vi "recursive2.vi"() -> ()   [LabVIEW 2014]
uses:
  <vilib>/LabVIEW Targets/FPGA/cRIO/shared/nicrio_ModuleControls/nicrio_cRIO-9467_Altitude.ctl
  <vilib>/LabVIEW Targets/FPGA/cRIO/shared/nicrio_ModuleControls/nicrio_cRIO-9467_Longitude.ctl
  <vilib>/LabVIEW Targets/FPGA/cRIO/shared/nicrio_ModuleControls/nicrio_cRIO-9467_Latitude.ctl
  <vilib>/LabVIEW Targets/FPGA/cRIO/shared/nicrio_ModuleControls/nicrio_cRIO-9225_DataRatesRing.ctl
  <vilib>/LabVIEW Targets/FPGA/cRIO/shared/nicrio_ModuleControls/nicrio_cRIO-9227_DataRatesRing.ctl
  <vilib>/rvi/FXPMathLib/FxpSinAndCos/subVIs/nifxpmath_SinAndCos_SimConfig.ctl
  <vilib>/rvi/FXPMathLib/FxpRectToPolar/subVIs/nifxpmath_RectToPolar_SimConfig.ctl
  <vilib>/rvi/Emulation/niFpgaGetClockAttributes.vi
  <vilib>/rvi/Emulation/niFpgaSctlEmulationGetInTimedLoop.vi
  <vilib>/rvi/Emulation/niFpgaEmulationReportErrorSimple.vi
  <vilib>/rvi/eio/common/nirviEmuTemplateMethod_errors.vi
  <vilib>/rvi/eio/common/nirviEmuTemplatePropertyGet_noerrors.vi
  <vilib>/rvi/Emulation/niFpgaCriticalErrorInLSC.vi
  <vilib>/rvi/Memory/Memory_Emulation/nirvimemoryFastEmulation.vi
  <vilib>/rvi/Memory/Memory_Emulation/nirvimemoryEmulation.vi
  <vilib>/rvi/Emulation/niFpgaEmulationIsFPGAContextNoSignature.vi
  <vilib>/rvi/DataTransferAndStorage/Container/Common/niFpgaContainerGetUniqueNameForEmu.vi
  <vilib>/rvi/Emulation/niFpgaProcessEmulError.vi
  <vilib>/rvi/errors/nirviReportUnexpectedCaseInternalError (U32).vi
  <vilib>/rvi/FXPMathLib/FxpSinAndCos/simVIs/DllFxpSinAndCosTemp_sub.vi
  <vilib>/rvi/FXPMathLib/FxpRectToPolar/simVIs/DllFxpRectToPolarTemp_sub.vi
  <vilib>/rvi/eio/common/nirviEmuTemplatePropertySet_noerrors.vi
  <vilib>/rvi/DataTransferAndStorage/Container/Common/niFpgaContainerSetEmuInfo.vi
  <vilib>/rvi/eio/common/nirviEmuReportErrorAndStop.vi
  <vilib>/rvi/eio/common/nirviEmuTemplatePropertyGet_errors.vi
  <vilib>/eio/EIOMethodNode/EIOMethodNode.xnode
  <vilib>/eio/EIOPropertyNode/EIOPropertyNode.xnode
  <vilib>/eio/EIONode/EIONode.xnode
  <vilib>/rvi/DataTransferAndStorage/Container/XNode/niFpgaContainer.xnode
  <vilib>/rvi/FXPMathLib/FxpMul/XNode/nifxpmath_Multiplier.xnode
  <vilib>/rvi/FXPMathLib/FxpSinAndCos/XNode/nifxpmath_SinAndCos.xnode
  <vilib>/rvi/FXPMathLib/FxpAdd/XNode/nifxpmath_Add.xnode
  <vilib>/rvi/FXPMathLib/FxpRectToPolar/XNode/nifxpmath_RectToPolar.xnode
  <vilib>/rvi/FXPMathLib/FxpSub/XNode/nifxpmath_Sub.xnode
  <vilib>/rvi/LocalResourceManager/LocalResourceManager.xnode
  <vilib>/rvi/FXPMathLib/sim/FxpSim.dll
  <vilib>/rvi/eio/common/nirviEmuTemplatePropertySet_errors.vi
  fpga timekeeper/FPGA Timekeeper.lvlib
panel:
  out "FPGA Timekeeper time (ns) 2":u64
  out "GPS status":T1(ring)
  out "FPGA Timekeeper locked":bool
  out "offset from time reference":i32
  out "antenna status":T2(ring)
  out "satellites available":u8
  out "UTC offset":i8
  out "UTC offset valid":bool
  out "Firmware Version":u32 format="%.0x"
  out "Vendor ID":u16 format="%.0x"
  out "Module ID":u16 format="%.0x"
  out "Serial Number":u32 format="%.0x"
  out "FPGA Error Out":errorcluster
  in  "stop 2":bool
  out "PPS Timestamp (TAI)":u64
  out "UTC Offset":i8
  out "UTC Offset Valid":bool
  out "GPS Status":T1(ring)
  out "Antenna Status":T2(ring)
  out "Leap Second Direction":enum8{"Add", "Delete"}(ring)
  out "Leap Second Pending":bool
  out "Leap Second Occurred":bool
  out "Satellites Available":u8
  out "Self-Survey Complete":bool
  out "Latitude (°)":T3 format="%.6f"
  out "Longitude (°)":T4 format="%.6g"
  out "Altitude (m)":T5 format="%.2f"
  out "Timed Out":bool
  out "Iterations":i32
  out "ROCOF":fxp<+/-,17,17>
  out "current frequency":fxp<+/-,35,18>
  out "Voltage Frequency":fxp<+/-,35,18>
  out "magnitude":fxp<+,62,19>[](array[numeric])
  out "phase angle":fxp<+/-,22,10>[](array[numeric])
  out "Array":T6(array[cluster])
  out "r":fxp<+,60,17>[](array[numeric])
  out "theta":fxp<+/-,22,10>[](array[numeric])
  in  "stop":bool
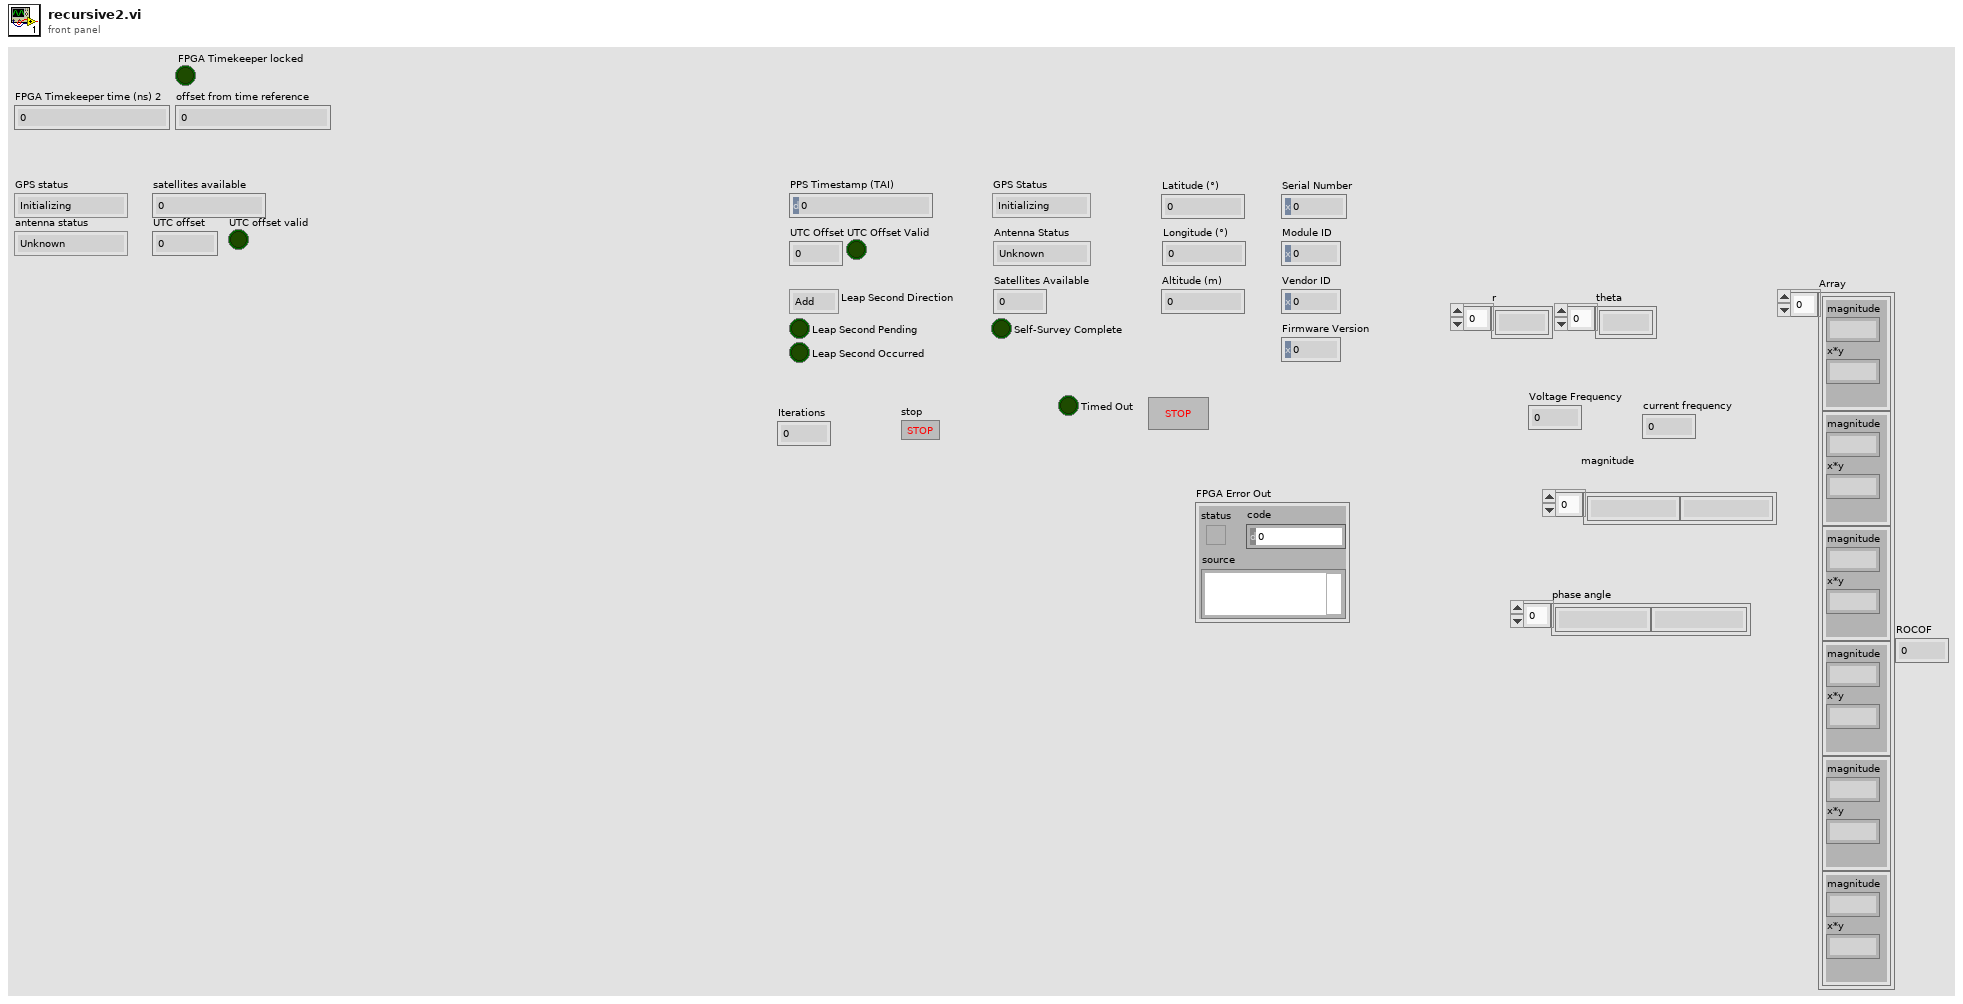
[diagram p1: front panel]
types:
  T1 = enum8{"Initializing", "Normal", "Unable to get fix"}
  T2 = enum8{"Unknown", "Normal", "Absent", "Overcurrent"}
  T3 = typedef "nicrio_cRIO-9467_Latitude.ctl" = fxp<+/-,28,8>
  T4 = typedef "nicrio_cRIO-9467_Longitude.ctl" = fxp<+/-,29,9>
  T5 = typedef "nicrio_cRIO-9467_Altitude.ctl" = fxp<+/-,24,17>
  T6 = cluster{"magnitude":fxp<+,62,19>, "x*y":fxp<+/-,22,10>}[]
  T7 = typedef "nicrio_cRIO-9227_DataRatesRing.ctl" = u8
  T8 = typedef "nicrio_cRIO-9225_DataRatesRing.ctl" = u8
  T9 = cluster{"magnitude":fxp<+,62,19>, "x*y":fxp<+/-,22,10>}
  T10 = cluster{"magnitude":fxp<+,60,17>, "x*y":fxp<+/-,22,10>}
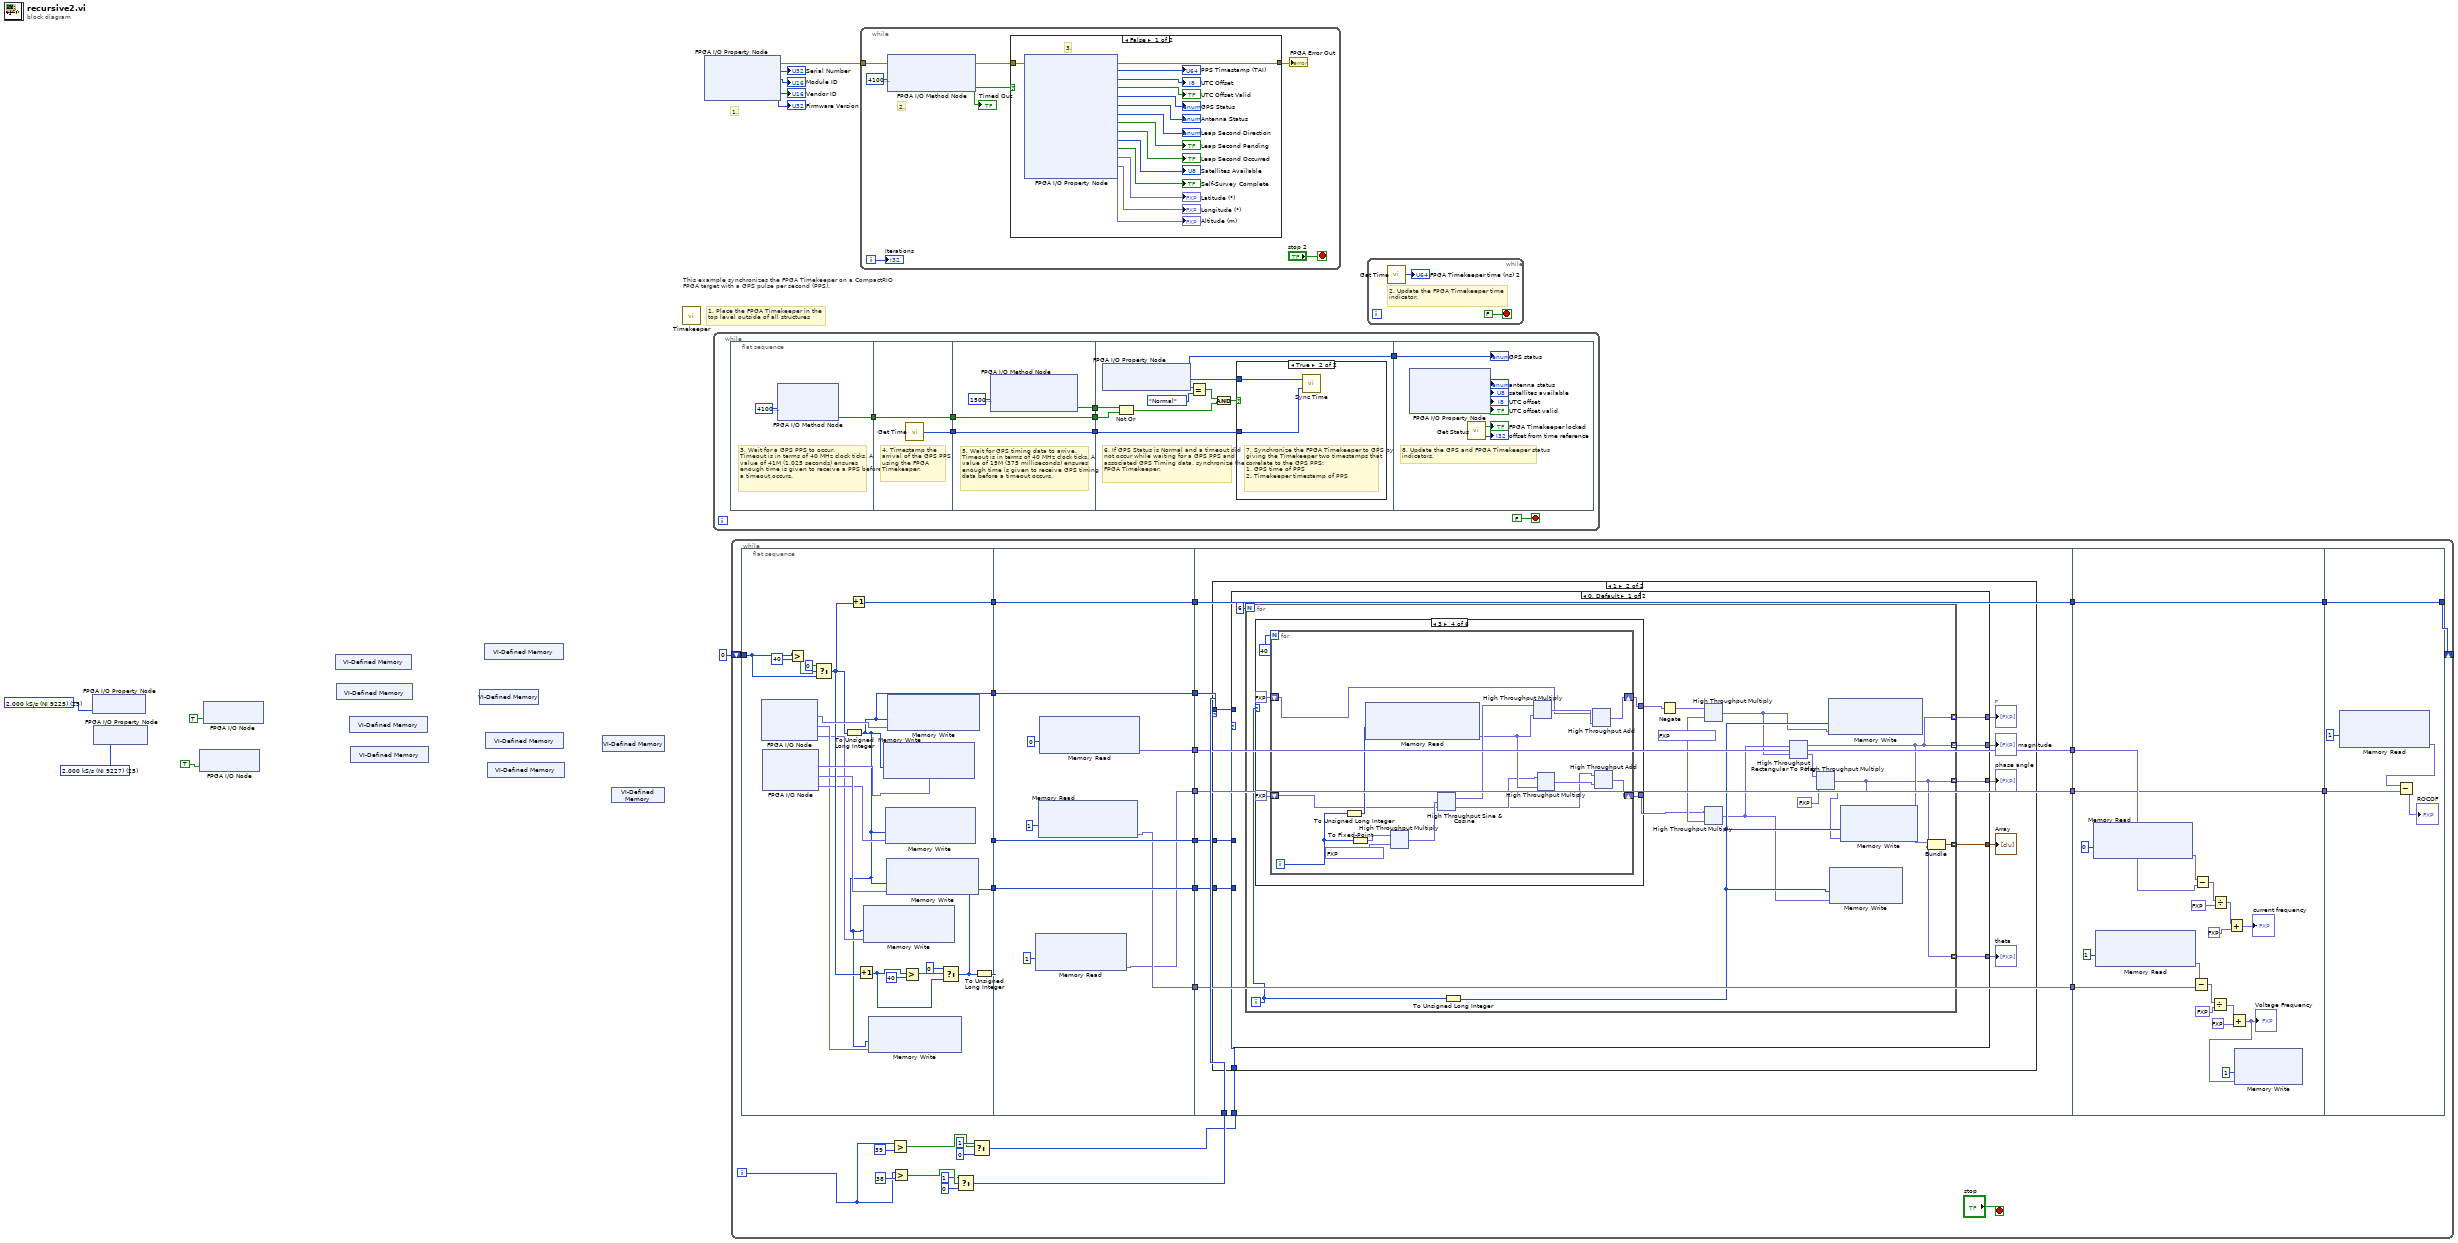
[diagram p0: block diagram]
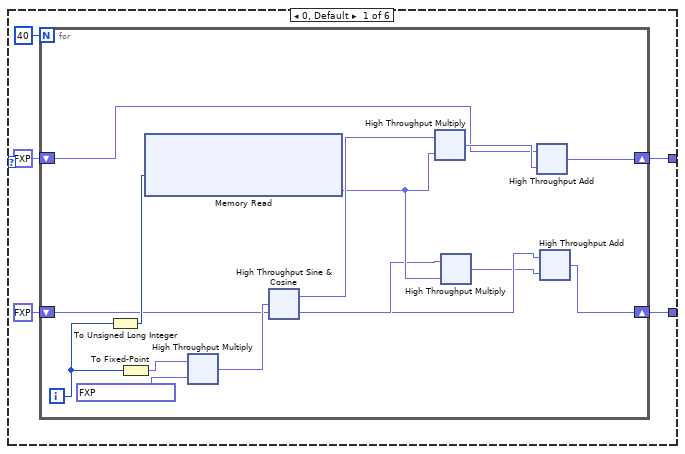
[diagram p5: hidden frame]
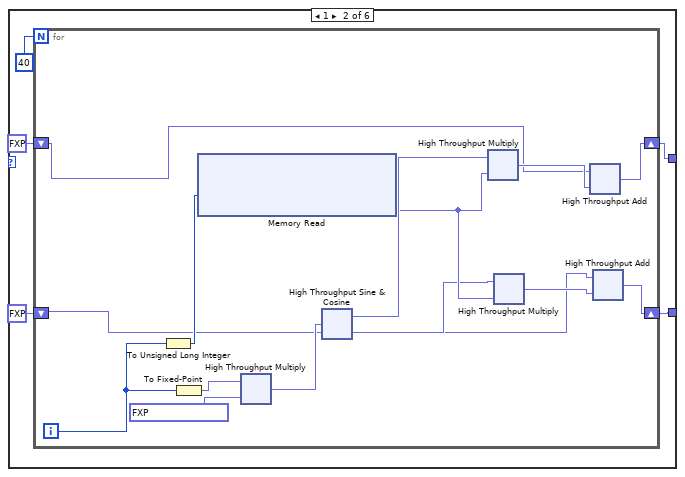
[diagram p6: hidden frame]
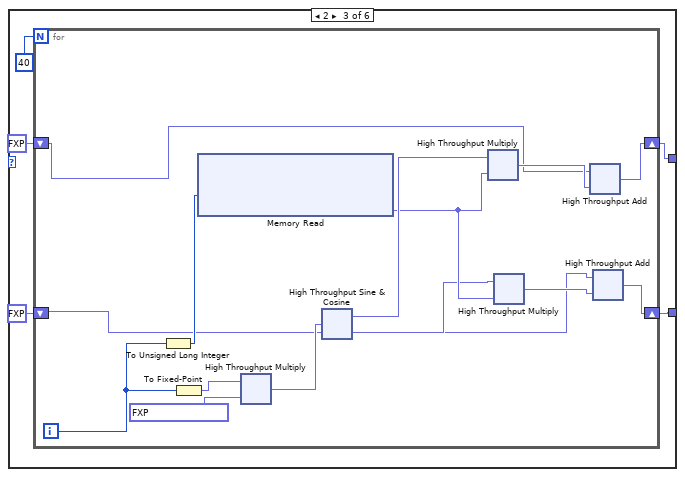
[diagram p7: hidden frame]
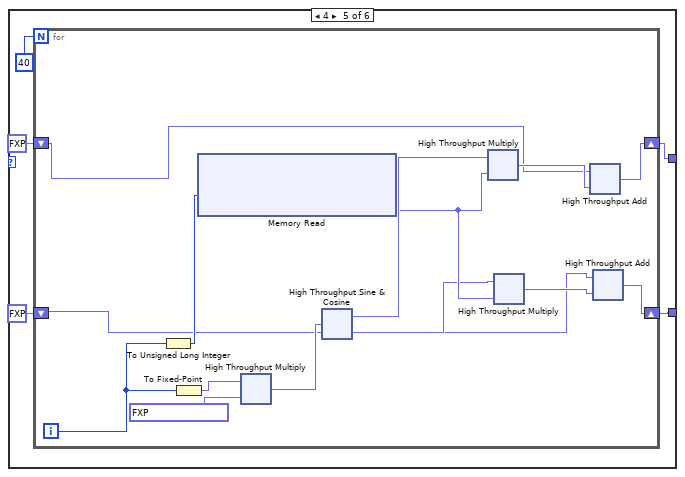
[diagram p8: hidden frame]
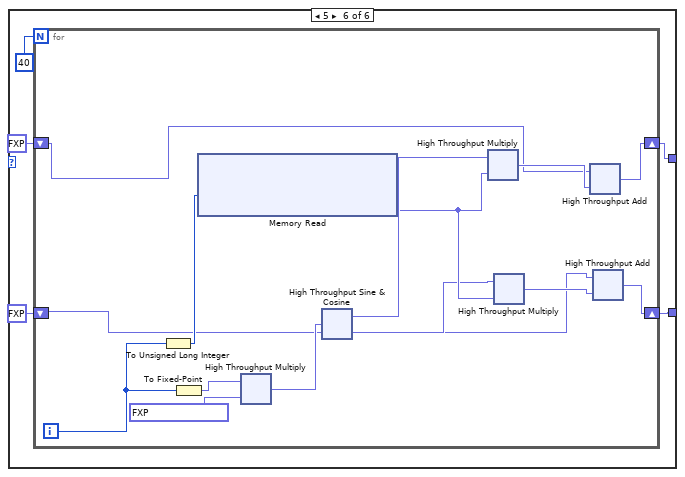
[diagram p9: hidden frame]
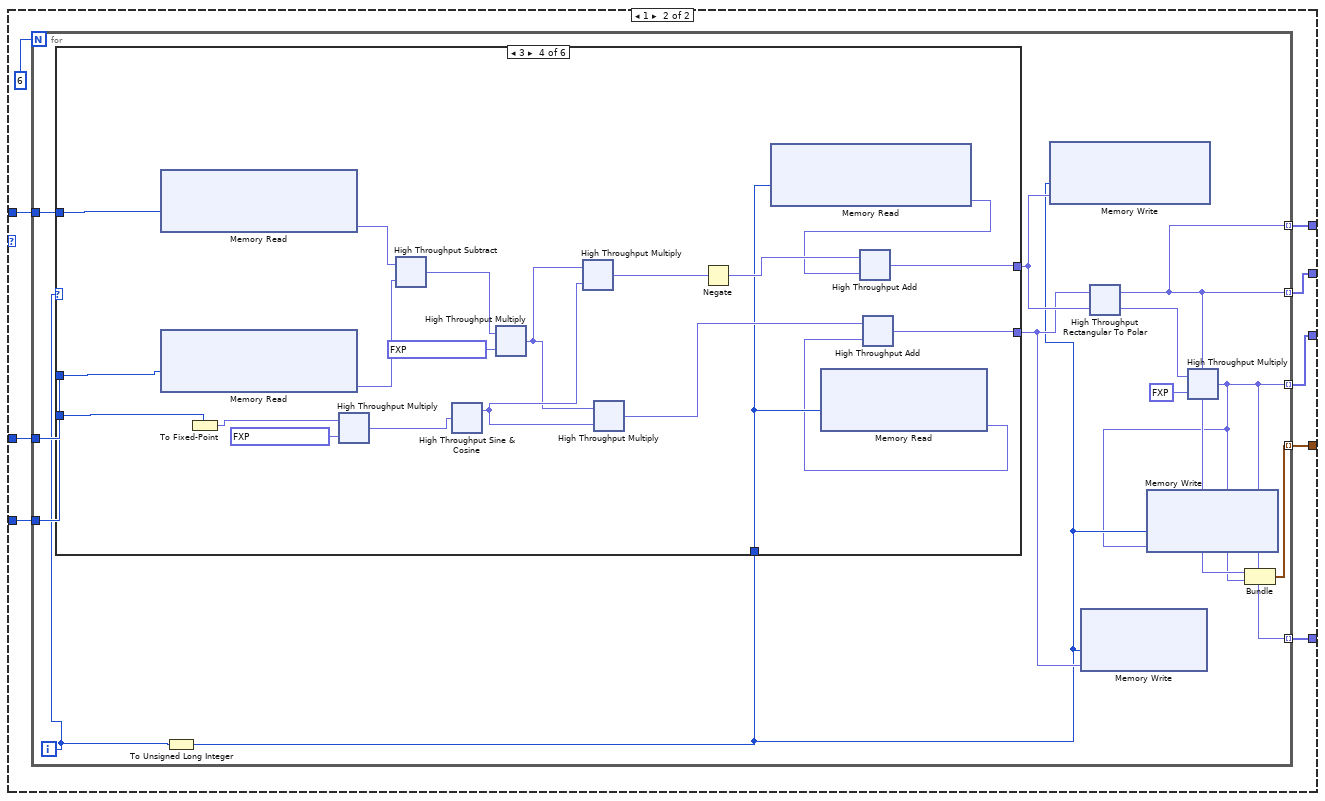
[diagram p10: hidden frame]
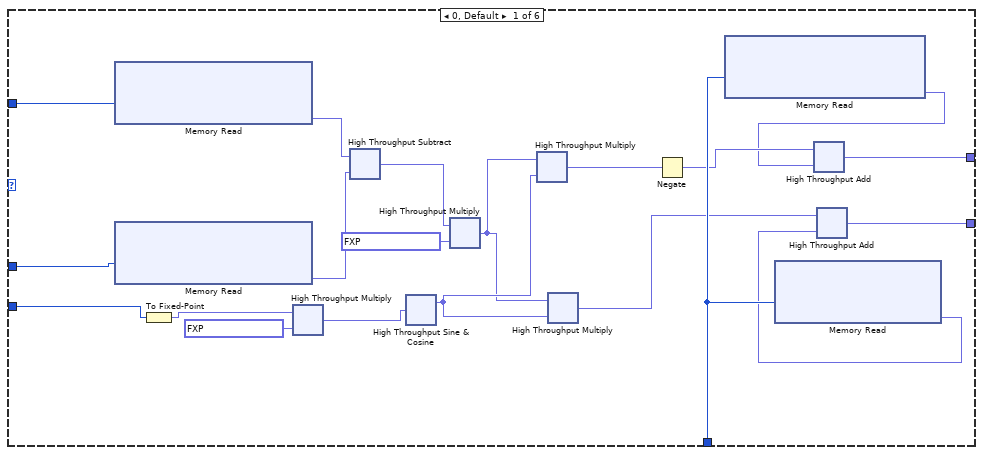
[diagram p11: hidden frame]
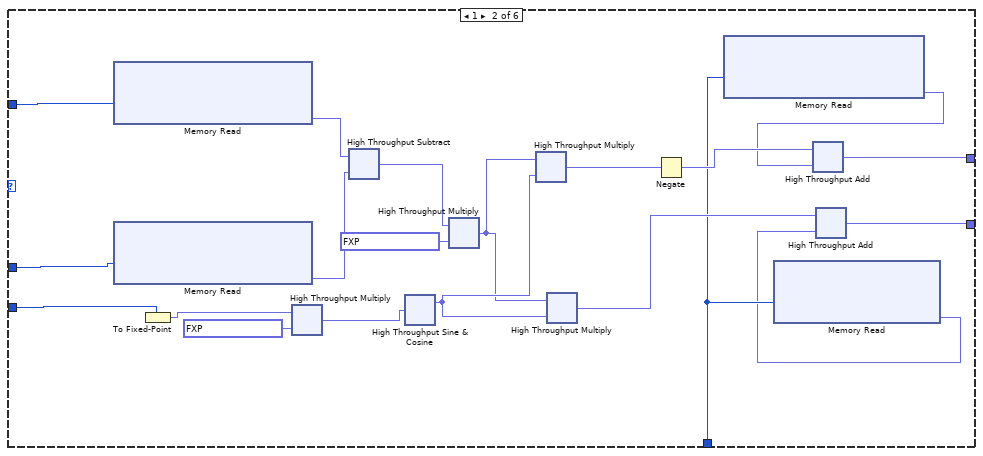
[diagram p12: hidden frame]
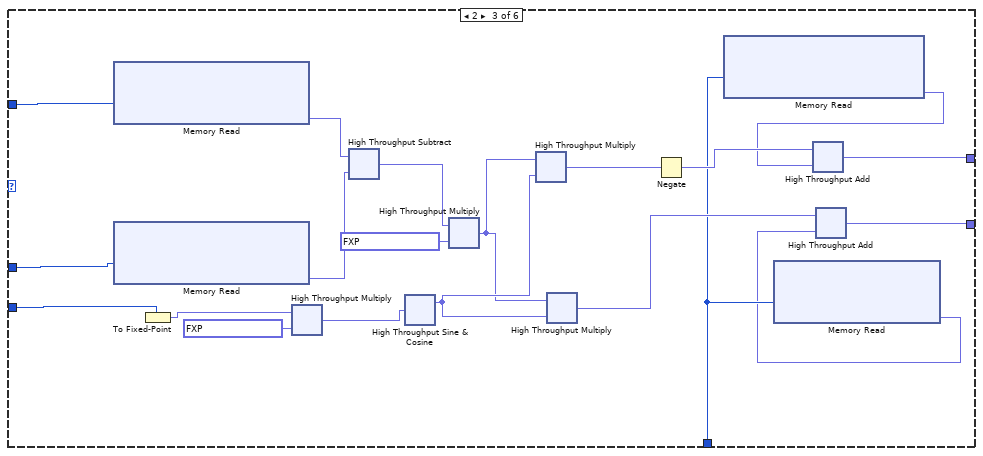
[diagram p13: hidden frame]
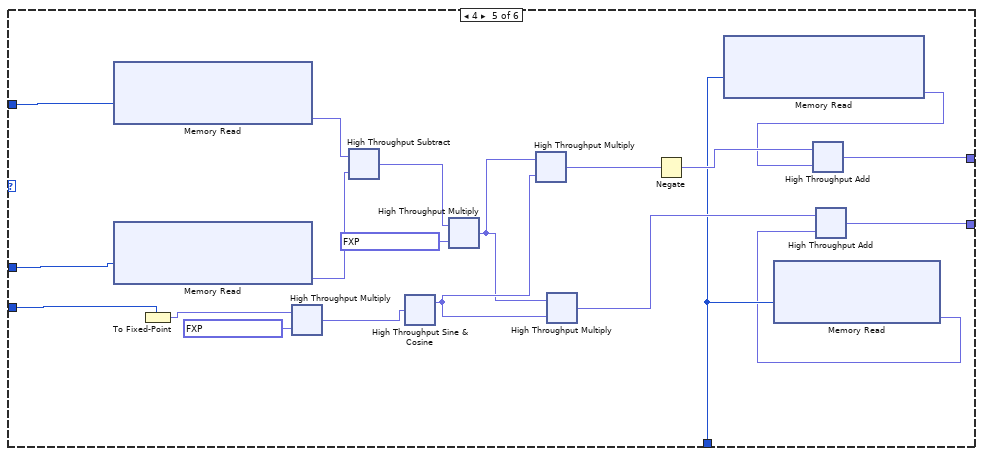
[diagram p14: hidden frame]
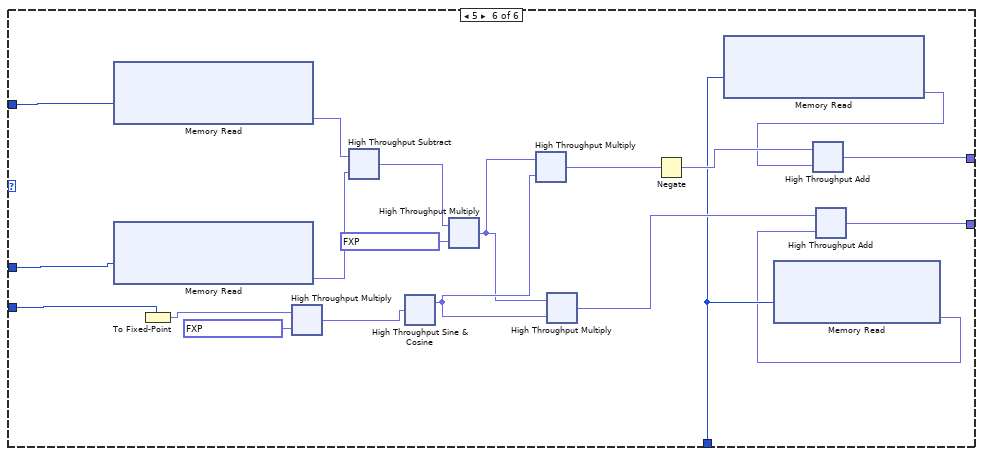
[diagram p15: hidden frame]
diagram:
  w10 = T7 25 items=["50.000 kS/s (NI 9227)"=1, "25.000 kS/s (NI 9227)"=2, "16.667 kS/s (NI 9227)"=3, "12.500 kS/s (NI 9227)"=4, "10.000 kS/s (NI 9227)"=5, "8.333 kS/s (NI 9227)"=6, "7.143 kS/s (NI 9227)"=7, "6.250 kS/s (NI 9227)"=8, "5.556 kS/s (NI 9227)"=9, "5.000 kS/s (NI 9227)"=10, "4.545 kS/s (NI 9227)"=11, "4.167 kS/s (NI 9227)"=12, "3.846 kS/s (NI 9227)"=13, "3.571 kS/s (NI 9227)"=14, "3.333 kS/s (NI 9227)"=15, "3.125 kS/s (NI 9227)"=16, "2.941 kS/s (NI 9227)"=17, "2.778 kS/s (NI 9227)"=18, "2.632 kS/s (NI 9227)"=19, "2.500 kS/s (NI 9227)"=20, "2.381 kS/s (NI 9227)"=21, "2.273 kS/s (NI 9227)"=22, "2.174 kS/s (NI 9227)"=23, "2.083 kS/s (NI 9227)"=24, "2.000 kS/s (NI 9227)"=25, "1.923 kS/s (NI 9227)"=26, "1.852 kS/s (NI 9227)"=27, "1.786 kS/s (NI 9227)"=28, "1.724 kS/s (NI 9227)"=29, "1.667 kS/s (NI 9227)"=30, "1.613 kS/s (NI 9227)"=31] ("Data Rate")
  w7 = T8 25 items=["50.000 kS/s (NI 9225)"=1, "25.000 kS/s (NI 9225)"=2, "16.667 kS/s (NI 9225)"=3, "12.500 kS/s (NI 9225)"=4, "10.000 kS/s (NI 9225)"=5, "8.333 kS/s (NI 9225)"=6, "7.143 kS/s (NI 9225)"=7, "6.250 kS/s (NI 9225)"=8, "5.556 kS/s (NI 9225)"=9, "5.000 kS/s (NI 9225)"=10, "4.545 kS/s (NI 9225)"=11, "4.167 kS/s (NI 9225)"=12, "3.846 kS/s (NI 9225)"=13, "3.571 kS/s (NI 9225)"=14, "3.333 kS/s (NI 9225)"=15, "3.125 kS/s (NI 9225)"=16, "2.941 kS/s (NI 9225)"=17, "2.778 kS/s (NI 9225)"=18, "2.632 kS/s (NI 9225)"=19, "2.500 kS/s (NI 9225)"=20, "2.381 kS/s (NI 9225)"=21, "2.273 kS/s (NI 9225)"=22, "2.174 kS/s (NI 9225)"=23, "2.083 kS/s (NI 9225)"=24, "2.000 kS/s (NI 9225)"=25, "1.923 kS/s (NI 9225)"=26, "1.852 kS/s (NI 9225)"=27, "1.786 kS/s (NI 9225)"=28, "1.724 kS/s (NI 9225)"=29, "1.667 kS/s (NI 9225)"=30, "1.613 kS/s (NI 9225)"=31] ("Data Rate")
  # "This example synchronizes the FPGA Timekeeper on a CompactRIO FPGA target with a GPS pulse per second (PPS)."
  # "1. Place the FPGA Timekeeper in the\ntop level outside of all structures"
  # "1."
  n1 = xnode "FPGA I/O Property Node"("Data Rate"=w7) -> ()  [unwired: 1 in, 1 out]
  n2 = xnode "FPGA I/O Property Node"("Data Rate"=w10) -> ()  [unwired: 1 in, 1 out]
  n3 = xnode "FPGA I/O Node"("Mod2/Start"=TRUE) -> ()  [unwired: 1 in, 1 out]
  n4 = xnode "FPGA I/O Node"("Mod1/Start"=TRUE) -> ()  [unwired: 1 in, 1 out]
  n5 = xnode "VI-Defined Memory"() -> ()  [unwired: 1 out]
  n6 = xnode "VI-Defined Memory"() -> ()  [unwired: 1 out]
  n7 = xnode "VI-Defined Memory"() -> ()  [unwired: 1 out]
  n8 = xnode "VI-Defined Memory"() -> ()  [unwired: 1 out]
  n9 = xnode "VI-Defined Memory"() -> ()  [unwired: 1 out]
  n10 = xnode "VI-Defined Memory"() -> ()  [unwired: 1 out]
  n11 = xnode "VI-Defined Memory"() -> ()  [unwired: 1 out]
  n12 = xnode "VI-Defined Memory"() -> ()  [unwired: 1 out]
  n13 = xnode "VI-Defined Memory"() -> ()  [unwired: 1 out]
  n14 = xnode "VI-Defined Memory"() -> ()  [unwired: 1 out]
  n15 = call "Timekeeper.vi"() -> ()  [unwired: 12 in]
  n16 = xnode "FPGA I/O Property Node"() -> ("error out"=w1:errorcluster, "Serial Number"=→"Serial Number":u32, "Module ID"=→"Module ID":u16, "Vendor ID"=→"Vendor ID":u16, "Firmware Version"=→"Firmware Version":u32)  [unwired: 2 in, 1 out]
  n17 = while {
    stop <- FALSE stop-if-true
    n18 = flat-sequence {
      tunnel: [w19] -> w17
      tunnel: w17 -> [w22]
      tunnel: [w22] -> w16
      tunnel: [w21] -> w14
      tunnel: [w25] -> w18
      tunnel: w16 -> [w24]
      tunnel: [w24] -> w15
      tunnel: w14 -> [w23]
      tunnel: [w23] -> w13
      tunnel: w18 -> [w34]
      tunnel: w15 -> [w33]
      tunnel: w13 -> [w28]
      tunnel: [w27] -> w12
      tunnel: w12 -> [w44]
      frame #0 {
        # "3. Wait for a GPS PPS to occur.\nTimeout is in terms of 40 MHz clock ticks. A value of 41M (1.025 seconds) ensures enough time is given to receive a PPS before a timeout occurs."
        n19 = xnode "FPGA I/O Method Node"("Timeout"=41000000) -> ("Timed Out"=w19:bool)  [unwired: 1 in, 1 out]
      }
      frame #1 {
        # "4. Timestamp the arrival of the GPS PPS using the FPGA Timekeeper."
        n20 = call "Get Time.vi"() -> ("time (ns)"=w21:u64)
      }
      frame #2 {
        # "5. Wait for GPS timing data to arrive.\nTimeout is in terms of 40 MHz clock ticks. A value of 15M (375 milliseconds) ensures enough time is given to receive GPS timing data before a timeout occurs."
        n21 = xnode "FPGA I/O Method Node"("Timeout"=15000000) -> ("Timed Out"=w25:bool)  [unwired: 1 in, 1 out]
      }
      frame #3 {
        # "6. If GPS Status is Normal and a timeout did not occur while waiting for a GPS PPS and associated GPS Timing data, synchronize the FPGA Timekeeper."
        n22 = xnode "FPGA I/O Property Node"() -> ("PPS Timestamp (TAI)"=w29:u64, "GPS Status"=w27:T1)  [unwired: 1 in, 1 out]
        n23 = Not Or(1:w33, 2:w34) -> (0:w31:bool)
        n24 = Equal?(x=w27, y=T1."Normal") -> (x = y?=w32:bool)
        n25 = And(x=w32, y=w31) -> (x .and. y?=w30:bool)
        n26 = case shown="True" w30 {
          tunnel: w29 -> [_ w37]
          tunnel: w28 -> [_ w36]
          frame False {
          }
          frame True {
            # "7. Synchronize the FPGA Timekeeper to GPS by giving the Timekeeper two timestamps that correlate to the GPS PPS:\n1. GPS time of PPS\n2. Timekeeper timestamp of PPS"
            n27 = call "Sync Time.vi"("FPGA Timekeeper time (ns)"=w36, "time reference time (ns)"=w37) -> ()
          }
        }
      }
      frame #4 {
        # "8. Update the GPS and FPGA Timekeeper status indicators."
        n28 = xnode "FPGA I/O Property Node"() -> ("Antenna Status"=→"antenna status":T2, "Satellites Available"=→"satellites available":u8, "UTC Offset"=→"UTC offset":i8, "UTC Offset Valid"=→"UTC offset valid":bool)  [unwired: 1 in, 1 out]
        n29 = call "Get Status.vi"() -> ("FPGA Timekeeper locked"=→"FPGA Timekeeper locked":bool, "offset from time reference"=→"offset from time reference":i32)
        "GPS status" <- w44
      }
    }
  }
  n30 = while {
    shift-right: [w74] -> _
    shift-left: i16 0 -> [w75]
    i -> [w64]
    stop <- "stop" stop-if-true
    n31 = flat-sequence {
      tunnel: w75 -> [w90]
      tunnel: [w89] -> w60
      tunnel: [w76] -> w58
      tunnel: [w82] -> w56
      tunnel: [w81] -> w54
      tunnel: w60 -> [w104]
      tunnel: [w104] -> w59
      tunnel: w58 -> [w103]
      tunnel: [w103] -> w57
      tunnel: w56 -> [w102]
      tunnel: [w102] -> w55
      tunnel: w54 -> [w101]
      tunnel: [w101] -> w53
      tunnel: [w98] -> w51
      tunnel: [w97] -> w50
      tunnel: [w95] -> w47
      tunnel: w59 -> [w113]
      tunnel: w70 -> [w112]
      tunnel: w67 -> [w111]
      tunnel: w57 -> [w110]
      tunnel: w55 -> [w109]
      tunnel: w53 -> [w108]
      tunnel: [w113] -> w61
      tunnel: [w107] -> w52
      tunnel: w51 -> [w107]
      tunnel: w50 -> [w106]
      tunnel: [w106] -> w49
      tunnel: w47 -> [w105]
      tunnel: [w105] -> w46
      tunnel: w61 -> [w849]
      tunnel: w52 -> [w844]
      tunnel: w49 -> [w843]
      tunnel: [w849] -> w48
      tunnel: w46 -> [w831]
      tunnel: [w831] -> w45
      tunnel: [w854] -> w74
      tunnel: w48 -> [w854]
      tunnel: w45 -> [w851]
      frame #0 {
        n32 = xnode "FPGA I/O Node"() -> ("Mod1/AI1"=w94:fxp<+/-,24,10>, "Mod1/AI2"=w78:fxp<+/-,24,10>, "Mod1/AI0"=w77:fxp<+/-,24,10>)  [unwired: 3 in, 3 out]
        n33 = xnode "FPGA I/O Node"() -> ("Mod2/AI1"=w93:fxp<+/-,24,5>, "Mod2/AI2"=w80:fxp<+/-,24,5>, "Mod2/AI0"=w79:fxp<+/-,24,5>)  [unwired: 3 in, 3 out]
        n34 = Greater?(x=w90, y=i16 40) -> (0:w91:bool)
        n35 = Select(t=i16 0, s=w91, f=w90) -> (s? t:f=w87:i16)
        n36 = To Unsigned Long Integer(number=w87) -> (unsigned 32bit integer=w76:u32)
        n37 = Increment(x=w87) -> (x+1=w89:i16)
        n38 = Increment(x=w87) -> (x+1=w84:i16)
        n39 = xnode ("Memory Write")("Address"=w76, "Data"=w77) -> ()  [unwired: 1 in, 1 out]
        n40 = xnode ("Memory Write")("Address"=w76, "Data"=w78) -> ()  [unwired: 1 in, 1 out]
        n41 = xnode ("Memory Write")("Address"=w76, "Data"=w93) -> ()  [unwired: 1 in, 1 out]
        n42 = xnode ("Memory Write")("Address"=w76, "Data"=w79) -> ()  [unwired: 1 in, 1 out]
        n43 = xnode ("Memory Write")("Address"=w76, "Data"=w80) -> ()  [unwired: 1 in, 1 out]
        n44 = xnode ("Memory Write")("Address"=w76, "Data"=w94) -> ()  [unwired: 1 in, 1 out]
        n45 = Greater?(x=w84, y=i16 40) -> (0:w85:bool)
        n46 = Select(t=i16 0, s=w85, f=w84) -> (s? t:f=w81:i16)
        n47 = To Unsigned Long Integer(number=w81) -> (unsigned 32bit integer=w82:u32)
      }
      frame #1 {
        n48 = xnode "Memory Read"("Address"=u32 1) -> ("Data"=w95:fxp<+/-,16,16>)  [unwired: 1 in, 1 out]
        n49 = xnode "Memory Read"("Address"=u32 1) -> ("Data"=w97:fxp<+/-,16,16>)  [unwired: 1 in, 1 out]
        n50 = xnode "Memory Read"("Address"=u32 0) -> ("Data"=w98:fxp<+/-,16,16>)  [unwired: 1 in, 1 out]
      }
      frame #2 {
        n51 = case shown="1" w112 {
          tunnel: w111 -> [_ w122]
          tunnel: w110 -> [_ w119]
          tunnel: w109 -> [_ w118]
          tunnel: w108 -> [_ w117]
          frame 0, Default {
          }
          frame 1 {
            n52 = case shown="0, Default" w122 {
              tunnel: [w127 w476] -> w121
              tunnel: [w126 w477] -> w120
              tunnel: w119 -> [_ w480]
              tunnel: w118 -> [_ w479]
              tunnel: w117 -> [_ w478]
              tunnel: [w125 w475] -> w116
              tunnel: [w124 w474] -> w115
              tunnel: [w123 w473] -> w114
              frame 0, Default {
                n53 = for {
                  N: 6 -> [_]
                  tunnel: [w132] -> w127 mode=indexing
                  tunnel: [w131] -> w126 mode=indexing
                  tunnel: [w133] -> w125 mode=indexing
                  tunnel: [w132] -> w124 mode=indexing
                  tunnel: [w131] -> w123 mode=indexing
                  i -> [w135]
                  w140 = fxp<+/-,16,1> 0.03533935546875 ("y")
                  n54 = case shown="3" w135 {
                    tunnel: [w181 w229 w278 w327 w376 w425] -> w137
                    tunnel: [w180 w228 w277 w326 w375 w424] -> w136
                    frame 0, Default {
                      n55 = for {
                        N: 40 -> [_]
                        shift-right: [w188] -> w181
                        shift-left: fxp<+,1,1> 0.0 -> [w187]
                        shift-right: [w184] -> w180
                        shift-left: fxp<+,1,1> 0.0 -> [w186]
                        i -> [w196]
                        n56 = To Unsigned Long Integer(number=w196) -> (unsigned 32bit integer=w197:u32)
                        n57 = To Fixed-Point(number=w196) -> (fixed-point=w195:fxp<+/-,32,32>)  [unwired: 1 in]
                        n58 = xnode ("Memory Read")("Address"=w197) -> ("Data"=w191:fxp<+/-,25,11>)  [unwired: 1 in, 1 out]
                        n59 = xnode ("High Throughput Multiply")("x"=w195, "y"=fxp<+/-,16,1> 0.04998779296875) -> ("x*y"=w193:fxp<+/-,48,33>)
                        n60 = xnode "High Throughput Sine & Cosine"("x (pi)"=w193) -> ("sin(x)"=w192:fxp<+/-,16,2>, "cos(x)"=w190:fxp<+/-,16,2>)
                        n61 = xnode ("High Throughput Multiply")("x"=w192, "y"=w191) -> ("x*y"=w189:fxp<+/-,41,13>)
                        n62 = xnode ("High Throughput Multiply")("x"=w190, "y"=w191) -> ("x*y"=w185:fxp<+/-,41,13>)
                        n63 = xnode ("High Throughput Add")("x"=w187, "y"=w189) -> ("x+y"=w188:fxp<+/-,45,17>)
                        n64 = xnode ("High Throughput Add")("x"=w186, "y"=w185) -> ("x+y"=w184:fxp<+/-,44,16>)
                      }
                    }
                    frame 1 {
                      n65 = for {
                        N: 40 -> [_]
                        shift-right: [w236] -> w229
                        shift-left: fxp<+/-,45,17> 0.0 ("x+y") -> [w235]
                        shift-right: [w237] -> w228
                        shift-left: fxp<+/-,44,16> 0.0 ("x+y") -> [w234]
                        i -> [w233]
                        n66 = To Unsigned Long Integer(number=w233) -> (unsigned 32bit integer=w246:u32)
                        n67 = To Fixed-Point(number=w233) -> (fixed-point=w245:fxp<+/-,32,32>)  [unwired: 1 in]
                        n68 = xnode ("Memory Read")("Address"=w246) -> ("Data"=w241:fxp<+/-,25,11>)  [unwired: 1 in, 1 out]
                        n69 = xnode ("High Throughput Multiply")("x"=w245, "y"=fxp<+/-,16,1> 0.04998779296875) -> ("x*y"=w243:fxp<+/-,48,33>)
                        n70 = xnode "High Throughput Sine & Cosine"("x (pi)"=w243) -> ("sin(x)"=w242:fxp<+/-,16,2>, "cos(x)"=w240:fxp<+/-,16,2>)
                        n71 = xnode ("High Throughput Multiply")("x"=w242, "y"=w241) -> ("x*y"=w239:fxp<+/-,41,13>)
                        n72 = xnode ("High Throughput Multiply")("x"=w240, "y"=w241) -> ("x*y"=w238:fxp<+/-,41,13>)
                        n73 = xnode ("High Throughput Add")("x"=w235, "y"=w239) -> ("x+y"=w236:fxp<+/-,45,17>)
                        n74 = xnode ("High Throughput Add")("x"=w234, "y"=w238) -> ("x+y"=w237:fxp<+/-,44,16>)
                      }
                    }
                    frame 2 {
                      n75 = for {
                        N: 40 -> [_]
                        shift-right: [w285] -> w278
                        shift-left: fxp<+/-,45,17> 0.0 ("x+y") -> [w284]
                        shift-right: [w286] -> w277
                        shift-left: fxp<+/-,44,16> 0.0 ("x+y") -> [w283]
                        i -> [w282]
                        n76 = To Unsigned Long Integer(number=w282) -> (unsigned 32bit integer=w295:u32)
                        n77 = To Fixed-Point(number=w282) -> (fixed-point=w294:fxp<+/-,32,32>)  [unwired: 1 in]
                        n78 = xnode ("Memory Read")("Address"=w295) -> ("Data"=w290:fxp<+/-,25,11>)  [unwired: 1 in, 1 out]
                        n79 = xnode ("High Throughput Multiply")("x"=w294, "y"=fxp<+/-,16,1> 0.04998779296875) -> ("x*y"=w292:fxp<+/-,48,33>)
                        n80 = xnode "High Throughput Sine & Cosine"("x (pi)"=w292) -> ("sin(x)"=w291:fxp<+/-,16,2>, "cos(x)"=w289:fxp<+/-,16,2>)
                        n81 = xnode ("High Throughput Multiply")("x"=w291, "y"=w290) -> ("x*y"=w288:fxp<+/-,41,13>)
                        n82 = xnode ("High Throughput Multiply")("x"=w289, "y"=w290) -> ("x*y"=w287:fxp<+/-,41,13>)
                        n83 = xnode ("High Throughput Add")("x"=w284, "y"=w288) -> ("x+y"=w285:fxp<+/-,45,17>)
                        n84 = xnode ("High Throughput Add")("x"=w283, "y"=w287) -> ("x+y"=w286:fxp<+/-,44,16>)
                      }
                    }
                    frame 3 {
                      n85 = for {
                        N: 40 -> [_]
                        shift-right: [w334] -> w327
                        shift-left: fxp<+/-,45,17> 0.0 ("x+y") -> [w333]
                        shift-right: [w335] -> w326
                        shift-left: fxp<+/-,44,16> 0.0 ("x+y") -> [w332]
                        i -> [w331]
                        n86 = To Unsigned Long Integer(number=w331) -> (unsigned 32bit integer=w344:u32)
                        n87 = To Fixed-Point(number=w331) -> (fixed-point=w343:fxp<+/-,32,32>)  [unwired: 1 in]
                        n88 = xnode ("Memory Read")("Address"=w344) -> ("Data"=w339:fxp<+/-,25,11>)  [unwired: 1 in, 1 out]
                        n89 = xnode ("High Throughput Multiply")("x"=w343, "y"=fxp<+/-,16,1> 0.04998779296875) -> ("x*y"=w341:fxp<+/-,48,33>)
                        n90 = xnode "High Throughput Sine & Cosine"("x (pi)"=w341) -> ("sin(x)"=w340:fxp<+/-,16,2>, "cos(x)"=w338:fxp<+/-,16,2>)
                        n91 = xnode ("High Throughput Multiply")("x"=w340, "y"=w339) -> ("x*y"=w337:fxp<+/-,41,13>)
                        n92 = xnode ("High Throughput Multiply")("x"=w338, "y"=w339) -> ("x*y"=w336:fxp<+/-,41,13>)
                        n93 = xnode ("High Throughput Add")("x"=w333, "y"=w337) -> ("x+y"=w334:fxp<+/-,45,17>)
                        n94 = xnode ("High Throughput Add")("x"=w332, "y"=w336) -> ("x+y"=w335:fxp<+/-,44,16>)
                      }
                    }
                    frame 4 {
                      n95 = for {
                        N: 40 -> [_]
                        shift-right: [w383] -> w376
                        shift-left: fxp<+/-,45,17> 0.0 ("x+y") -> [w382]
                        shift-right: [w384] -> w375
                        shift-left: fxp<+/-,44,16> 0.0 ("x+y") -> [w381]
                        i -> [w380]
                        n96 = To Unsigned Long Integer(number=w380) -> (unsigned 32bit integer=w393:u32)
                        n97 = To Fixed-Point(number=w380) -> (fixed-point=w392:fxp<+/-,32,32>)  [unwired: 1 in]
                        n98 = xnode ("Memory Read")("Address"=w393) -> ("Data"=w388:fxp<+/-,25,11>)  [unwired: 1 in, 1 out]
                        n99 = xnode ("High Throughput Multiply")("x"=w392, "y"=fxp<+/-,16,1> 0.04998779296875) -> ("x*y"=w390:fxp<+/-,48,33>)
                        n100 = xnode "High Throughput Sine & Cosine"("x (pi)"=w390) -> ("sin(x)"=w389:fxp<+/-,16,2>, "cos(x)"=w387:fxp<+/-,16,2>)
                        n101 = xnode ("High Throughput Multiply")("x"=w389, "y"=w388) -> ("x*y"=w386:fxp<+/-,41,13>)
                        n102 = xnode ("High Throughput Multiply")("x"=w387, "y"=w388) -> ("x*y"=w385:fxp<+/-,41,13>)
                        n103 = xnode ("High Throughput Add")("x"=w382, "y"=w386) -> ("x+y"=w383:fxp<+/-,45,17>)
                        n104 = xnode ("High Throughput Add")("x"=w381, "y"=w385) -> ("x+y"=w384:fxp<+/-,44,16>)
                      }
                    }
                    frame 5 {
                      n105 = for {
                        N: 40 -> [_]
                        shift-right: [w432] -> w425
                        shift-left: fxp<+/-,45,17> 0.0 ("x+y") -> [w431]
                        shift-right: [w433] -> w424
                        shift-left: fxp<+/-,44,16> 0.0 ("x+y") -> [w430]
                        i -> [w429]
                        n106 = To Unsigned Long Integer(number=w429) -> (unsigned 32bit integer=w442:u32)
                        n107 = To Fixed-Point(number=w429) -> (fixed-point=w441:fxp<+/-,32,32>)  [unwired: 1 in]
                        n108 = xnode ("Memory Read")("Address"=w442) -> ("Data"=w437:fxp<+/-,25,11>)  [unwired: 1 in, 1 out]
                        n109 = xnode ("High Throughput Multiply")("x"=w441, "y"=fxp<+/-,16,1> 0.04998779296875) -> ("x*y"=w439:fxp<+/-,48,33>)
                        n110 = xnode "High Throughput Sine & Cosine"("x (pi)"=w439) -> ("sin(x)"=w438:fxp<+/-,16,2>, "cos(x)"=w436:fxp<+/-,16,2>)
                        n111 = xnode ("High Throughput Multiply")("x"=w438, "y"=w437) -> ("x*y"=w435:fxp<+/-,41,13>)
                        n112 = xnode ("High Throughput Multiply")("x"=w436, "y"=w437) -> ("x*y"=w434:fxp<+/-,41,13>)
                        n113 = xnode ("High Throughput Add")("x"=w431, "y"=w435) -> ("x+y"=w432:fxp<+/-,45,17>)
                        n114 = xnode ("High Throughput Add")("x"=w430, "y"=w434) -> ("x+y"=w433:fxp<+/-,44,16>)
                      }
                    }
                  }
                  n115 = To Unsigned Long Integer(number=w135) -> (unsigned 32bit integer=w134:u32)
                  n116 = Negate(x=w137) -> (-x=w141:fxp<+/-,46,18>)
                  n117 = xnode ("High Throughput Multiply")("x"=w141, "y"=w140) -> ("x*y"=w129:fxp<+/-,62,19>)
                  n118 = xnode ("High Throughput Multiply")("x"=w136, "y"=w140) -> ("x*y"=w130:fxp<+/-,60,17>)
                  n119 = xnode "High Throughput Rectangular To Polar"("x"=w130, "y"=w129) -> ("magnitude"=w132:fxp<+,62,19>, "phase (pi)"=w139:fxp<+/-,16,2>)
                  n120 = xnode ("High Throughput Multiply")("x"=w139, "y"=fxp<+,6,8> 180.0) -> ("x*y"=w131:fxp<+/-,22,10>)
                  n121 = xnode ("Memory Write")("Address"=w134, "Data"=w129) -> ()  [unwired: 1 in, 1 out]
                  n122 = xnode ("Memory Write")("Address"=w134, "Data"=w130) -> ()  [unwired: 1 in, 1 out]
                  n123 = xnode "Memory Write"("Address"=w134, "Data"=w131) -> ()  [unwired: 1 in, 1 out]
                  n124 = Bundle("magnitude"=w132, "x*y"=w131) -> (w133:T9)  [unwired: 1 in]
                }
              }
              frame 1 {
                n125 = for {
                  N: 6 -> [_]
                  tunnel: w480 -> [w493]
                  tunnel: w479 -> [w492]
                  tunnel: w478 -> [w491]
                  tunnel: [w482] -> w477 mode=indexing
                  tunnel: [w483] -> w476 mode=indexing
                  tunnel: [w484] -> w475 mode=indexing
                  tunnel: [w483] -> w474 mode=indexing
                  tunnel: [w482] -> w473 mode=indexing
                  i -> [w490]
                  n126 = To Unsigned Long Integer(number=w490) -> (unsigned 32bit integer=w485:u32)
                  n127 = case shown="3" w490 {
                    tunnel: w493 -> [w550 w587 w637 w687 w737 w787]
                    tunnel: w492 -> [w549 w586 w636 w686 w736 w786]
                    tunnel: w491 -> [w544 w585 w635 w685 w735 w785]
                    tunnel: w485 -> [w538 w584 w634 w684 w734 w784]
                    tunnel: [w532 w581 w631 w681 w731 w781] -> w487
                    tunnel: [w531 w582 w632 w682 w732 w782] -> w486
                    frame 0, Default {
                      n128 = xnode ("Memory Read")("Address"=w550) -> ("Data"=w548:fxp<+/-,25,11>)  [unwired: 1 in, 1 out]
                      n129 = xnode ("Memory Read")("Address"=w549) -> ("Data"=w547:fxp<+/-,25,11>)  [unwired: 1 in, 1 out]
                      n130 = To Fixed-Point(number=w544) -> (fixed-point=w543:fxp<+/-,16,16>)  [unwired: 1 in]
                      n131 = xnode ("High Throughput Multiply")("x"=w543, "y"=fxp<+/-,16,1> 0.04998779296875) -> ("x*y"=w541:fxp<+/-,32,17>)
                      n132 = xnode "High Throughput Subtract"("x"=w548, "y"=w547) -> ("x-y"=w546:fxp<+/-,26,12>)
                      n133 = xnode "High Throughput Sine & Cosine"("x (pi)"=w541) -> ("sin(x)"=w540:fxp<+/-,16,2>)  [unwired: 1 out]
                      n134 = xnode ("High Throughput Multiply")("x"=w546, "y"=fxp<+/-,16,1> 0.03533935546875) -> ("x*y"=w539:fxp<+/-,42,13>)
                      n135 = xnode ("High Throughput Multiply")("x"=w539, "y"=w540) -> ("x*y"=w537:fxp<+/-,58,15>)
                      n136 = xnode ("High Throughput Multiply")("x"=w539, "y"=w540) -> ("x*y"=w533:fxp<+/-,58,15>)
                      n137 = Negate(x=w537) -> (-x=w536:fxp<+/-,59,16>)
                      n138 = xnode ("Memory Read")("Address"=w538) -> ("Data"=w535:fxp<+/-,25,11>)  [unwired: 1 in, 1 out]
                      n139 = xnode ("Memory Read")("Address"=w538) -> ("Data"=w534:fxp<+/-,25,11>)  [unwired: 1 in, 1 out]
                      n140 = xnode ("High Throughput Add")("x"=w536, "y"=w535) -> ("x+y"=w532:fxp<+/-,60,17>)
                      n141 = xnode ("High Throughput Add")("x"=w533, "y"=w534) -> ("x+y"=w531:fxp<+/-,59,16>)
                    }
                    frame 1 {
                      n142 = xnode ("Memory Read")("Address"=w587) -> ("Data"=w600:fxp<+/-,25,11>)  [unwired: 1 in, 1 out]
                      n143 = xnode ("Memory Read")("Address"=w586) -> ("Data"=w599:fxp<+/-,25,11>)  [unwired: 1 in, 1 out]
                      n144 = To Fixed-Point(number=w585) -> (fixed-point=w596:fxp<+/-,16,16>)  [unwired: 1 in]
                      n145 = xnode ("High Throughput Multiply")("x"=w596, "y"=fxp<+/-,16,1> 0.04998779296875) -> ("x*y"=w594:fxp<+/-,32,17>)
                      n146 = xnode "High Throughput Subtract"("x"=w600, "y"=w599) -> ("x-y"=w598:fxp<+/-,26,12>)
                      n147 = xnode "High Throughput Sine & Cosine"("x (pi)"=w594) -> ("sin(x)"=w593:fxp<+/-,16,2>)  [unwired: 1 out]
                      n148 = xnode ("High Throughput Multiply")("x"=w598, "y"=fxp<+/-,16,1> 0.03533935546875) -> ("x*y"=w592:fxp<+/-,42,13>)
                      n149 = xnode ("High Throughput Multiply")("x"=w592, "y"=w593) -> ("x*y"=w591:fxp<+/-,58,15>)
                      n150 = xnode ("High Throughput Multiply")("x"=w592, "y"=w593) -> ("x*y"=w588:fxp<+/-,58,15>)
                      n151 = Negate(x=w591) -> (-x=w590:fxp<+/-,59,16>)
                      n152 = xnode ("Memory Read")("Address"=w584) -> ("Data"=w589:fxp<+/-,25,11>)  [unwired: 1 in, 1 out]
                      n153 = xnode ("Memory Read")("Address"=w584) -> ("Data"=w583:fxp<+/-,25,11>)  [unwired: 1 in, 1 out]
                      n154 = xnode ("High Throughput Add")("x"=w590, "y"=w589) -> ("x+y"=w581:fxp<+/-,60,17>)
                      n155 = xnode ("High Throughput Add")("x"=w588, "y"=w583) -> ("x+y"=w582:fxp<+/-,59,16>)
                    }
                    frame 2 {
                      n156 = xnode ("Memory Read")("Address"=w637) -> ("Data"=w650:fxp<+/-,25,11>)  [unwired: 1 in, 1 out]
                      n157 = xnode ("Memory Read")("Address"=w636) -> ("Data"=w649:fxp<+/-,25,11>)  [unwired: 1 in, 1 out]
                      n158 = To Fixed-Point(number=w635) -> (fixed-point=w646:fxp<+/-,16,16>)  [unwired: 1 in]
                      n159 = xnode ("High Throughput Multiply")("x"=w646, "y"=fxp<+/-,16,1> 0.04998779296875) -> ("x*y"=w644:fxp<+/-,32,17>)
                      n160 = xnode "High Throughput Subtract"("x"=w650, "y"=w649) -> ("x-y"=w648:fxp<+/-,26,12>)
                      n161 = xnode "High Throughput Sine & Cosine"("x (pi)"=w644) -> ("sin(x)"=w643:fxp<+/-,16,2>)  [unwired: 1 out]
                      n162 = xnode ("High Throughput Multiply")("x"=w648, "y"=fxp<+/-,16,1> 0.03533935546875) -> ("x*y"=w642:fxp<+/-,42,13>)
                      n163 = xnode ("High Throughput Multiply")("x"=w642, "y"=w643) -> ("x*y"=w641:fxp<+/-,58,15>)
                      n164 = xnode ("High Throughput Multiply")("x"=w642, "y"=w643) -> ("x*y"=w638:fxp<+/-,58,15>)
                      n165 = Negate(x=w641) -> (-x=w640:fxp<+/-,59,16>)
                      n166 = xnode ("Memory Read")("Address"=w634) -> ("Data"=w639:fxp<+/-,25,11>)  [unwired: 1 in, 1 out]
                      n167 = xnode ("Memory Read")("Address"=w634) -> ("Data"=w633:fxp<+/-,25,11>)  [unwired: 1 in, 1 out]
                      n168 = xnode ("High Throughput Add")("x"=w640, "y"=w639) -> ("x+y"=w631:fxp<+/-,60,17>)
                      n169 = xnode ("High Throughput Add")("x"=w638, "y"=w633) -> ("x+y"=w632:fxp<+/-,59,16>)
                    }
                    frame 3 {
                      n170 = xnode ("Memory Read")("Address"=w687) -> ("Data"=w700:fxp<+/-,25,11>)  [unwired: 1 in, 1 out]
                      n171 = xnode ("Memory Read")("Address"=w686) -> ("Data"=w699:fxp<+/-,25,11>)  [unwired: 1 in, 1 out]
                      n172 = To Fixed-Point(number=w685) -> (fixed-point=w696:fxp<+/-,16,16>)  [unwired: 1 in]
                      n173 = xnode ("High Throughput Multiply")("x"=w696, "y"=fxp<+/-,16,1> 0.04998779296875) -> ("x*y"=w694:fxp<+/-,32,17>)
                      n174 = xnode "High Throughput Subtract"("x"=w700, "y"=w699) -> ("x-y"=w698:fxp<+/-,26,12>)
                      n175 = xnode "High Throughput Sine & Cosine"("x (pi)"=w694) -> ("sin(x)"=w693:fxp<+/-,16,2>)  [unwired: 1 out]
                      n176 = xnode ("High Throughput Multiply")("x"=w698, "y"=fxp<+/-,16,1> 0.03533935546875) -> ("x*y"=w692:fxp<+/-,42,13>)
                      n177 = xnode ("High Throughput Multiply")("x"=w692, "y"=w693) -> ("x*y"=w691:fxp<+/-,58,15>)
                      n178 = xnode ("High Throughput Multiply")("x"=w692, "y"=w693) -> ("x*y"=w688:fxp<+/-,58,15>)
                      n179 = Negate(x=w691) -> (-x=w690:fxp<+/-,59,16>)
                      n180 = xnode ("Memory Read")("Address"=w684) -> ("Data"=w689:fxp<+/-,25,11>)  [unwired: 1 in, 1 out]
                      n181 = xnode ("Memory Read")("Address"=w684) -> ("Data"=w683:fxp<+/-,25,11>)  [unwired: 1 in, 1 out]
                      n182 = xnode ("High Throughput Add")("x"=w690, "y"=w689) -> ("x+y"=w681:fxp<+/-,60,17>)
                      n183 = xnode ("High Throughput Add")("x"=w688, "y"=w683) -> ("x+y"=w682:fxp<+/-,59,16>)
                    }
                    frame 4 {
                      n184 = xnode ("Memory Read")("Address"=w737) -> ("Data"=w750:fxp<+/-,25,11>)  [unwired: 1 in, 1 out]
                      n185 = xnode ("Memory Read")("Address"=w736) -> ("Data"=w749:fxp<+/-,25,11>)  [unwired: 1 in, 1 out]
                      n186 = To Fixed-Point(number=w735) -> (fixed-point=w746:fxp<+/-,16,16>)  [unwired: 1 in]
                      n187 = xnode ("High Throughput Multiply")("x"=w746, "y"=fxp<+/-,16,1> 0.04998779296875) -> ("x*y"=w744:fxp<+/-,32,17>)
                      n188 = xnode "High Throughput Subtract"("x"=w750, "y"=w749) -> ("x-y"=w748:fxp<+/-,26,12>)
                      n189 = xnode "High Throughput Sine & Cosine"("x (pi)"=w744) -> ("sin(x)"=w743:fxp<+/-,16,2>)  [unwired: 1 out]
                      n190 = xnode ("High Throughput Multiply")("x"=w748, "y"=fxp<+/-,16,1> 0.03533935546875) -> ("x*y"=w742:fxp<+/-,42,13>)
                      n191 = xnode ("High Throughput Multiply")("x"=w742, "y"=w743) -> ("x*y"=w741:fxp<+/-,58,15>)
                      n192 = xnode ("High Throughput Multiply")("x"=w742, "y"=w743) -> ("x*y"=w738:fxp<+/-,58,15>)
                      n193 = Negate(x=w741) -> (-x=w740:fxp<+/-,59,16>)
                      n194 = xnode ("Memory Read")("Address"=w734) -> ("Data"=w739:fxp<+/-,25,11>)  [unwired: 1 in, 1 out]
                      n195 = xnode ("Memory Read")("Address"=w734) -> ("Data"=w733:fxp<+/-,25,11>)  [unwired: 1 in, 1 out]
                      n196 = xnode ("High Throughput Add")("x"=w740, "y"=w739) -> ("x+y"=w731:fxp<+/-,60,17>)
                      n197 = xnode ("High Throughput Add")("x"=w738, "y"=w733) -> ("x+y"=w732:fxp<+/-,59,16>)
                    }
                    frame 5 {
                      n198 = xnode ("Memory Read")("Address"=w787) -> ("Data"=w800:fxp<+/-,25,11>)  [unwired: 1 in, 1 out]
                      n199 = xnode ("Memory Read")("Address"=w786) -> ("Data"=w799:fxp<+/-,25,11>)  [unwired: 1 in, 1 out]
                      n200 = To Fixed-Point(number=w785) -> (fixed-point=w796:fxp<+/-,16,16>)  [unwired: 1 in]
                      n201 = xnode ("High Throughput Multiply")("x"=w796, "y"=fxp<+/-,16,1> 0.04998779296875) -> ("x*y"=w794:fxp<+/-,32,17>)
                      n202 = xnode "High Throughput Subtract"("x"=w800, "y"=w799) -> ("x-y"=w798:fxp<+/-,26,12>)
                      n203 = xnode "High Throughput Sine & Cosine"("x (pi)"=w794) -> ("sin(x)"=w793:fxp<+/-,16,2>)  [unwired: 1 out]
                      n204 = xnode ("High Throughput Multiply")("x"=w798, "y"=fxp<+/-,16,1> 0.03533935546875) -> ("x*y"=w792:fxp<+/-,42,13>)
                      n205 = xnode ("High Throughput Multiply")("x"=w792, "y"=w793) -> ("x*y"=w791:fxp<+/-,58,15>)
                      n206 = xnode ("High Throughput Multiply")("x"=w792, "y"=w793) -> ("x*y"=w788:fxp<+/-,58,15>)
                      n207 = Negate(x=w791) -> (-x=w790:fxp<+/-,59,16>)
                      n208 = xnode ("Memory Read")("Address"=w784) -> ("Data"=w789:fxp<+/-,25,11>)  [unwired: 1 in, 1 out]
                      n209 = xnode ("Memory Read")("Address"=w784) -> ("Data"=w783:fxp<+/-,25,11>)  [unwired: 1 in, 1 out]
                      n210 = xnode ("High Throughput Add")("x"=w790, "y"=w789) -> ("x+y"=w781:fxp<+/-,60,17>)
                      n211 = xnode ("High Throughput Add")("x"=w788, "y"=w783) -> ("x+y"=w782:fxp<+/-,59,16>)
                    }
                  }
                  n212 = xnode ("Memory Write")("Address"=w485, "Data"=w487) -> ()  [unwired: 1 in, 1 out]
                  n213 = xnode ("Memory Write")("Address"=w485, "Data"=w486) -> ()  [unwired: 1 in, 1 out]
                  n214 = xnode "High Throughput Rectangular To Polar"("x"=w486, "y"=w487) -> ("magnitude"=w483:fxp<+,60,17>, "phase (pi)"=w489:fxp<+/-,16,2>)
                  n215 = xnode ("High Throughput Multiply")("x"=w489, "y"=fxp<+,6,8> 180.0) -> ("x*y"=w482:fxp<+/-,22,10>)
                  n216 = xnode "Memory Write"("Address"=w485, "Data"=w482) -> ()  [unwired: 1 in, 1 out]
                  n217 = Bundle("magnitude"=w483, "x*y"=w482) -> (w484:T10)  [unwired: 1 in]
                }
              }
            }
            "magnitude" <- w121
            "phase angle" <- w120
            "Array" <- w116
            "r" <- w115
            "theta" <- w114
          }
        }
      }
      frame #3 {
        n218 = xnode "Memory Read"("Address"=u32 0) -> ("Data"=w847:fxp<+/-,16,16>)  [unwired: 1 in, 1 out]
        n219 = xnode "Memory Read"("Address"=u32 1) -> ("Data"=w848:fxp<+/-,16,16>)  [unwired: 1 in, 1 out]
        n220 = Subtract(x=w848, y=w843) -> (x-y=w841:fxp<+/-,17,17>)
        n221 = Subtract(x=w847, y=w844) -> (x-y=w842:fxp<+/-,17,17>)
        n222 = Divide(x=w841, y=fxp<+/-,17,17> 360.0) -> (x/y=w836:fxp<+/-,34,17>)
        n223 = Divide(x=w842, y=fxp<+/-,17,17> 360.0) -> (x/y=w835:fxp<+/-,34,17>)
        n224 = Add(x=w835, y=fxp<+,5,6> 50.0) -> (x+y=→"current frequency":fxp<+/-,35,18>)
        n225 = Add(x=w836, y=fxp<+,5,6> 50.0) -> (x+y=w832:fxp<+/-,35,18>)
        "Voltage Frequency" <- w832
        n226 = xnode "Memory Write"("Address"=u32 1, "Data"=w832) -> ()  [unwired: 1 in, 1 out]
      }
      frame #4 {
        n227 = xnode "Memory Read"("Address"=u32 1) -> ("Data"=w852:fxp<+/-,16,16>)  [unwired: 1 in, 1 out]
        n228 = Subtract(x=w852, y=w851) -> (x-y=→"ROCOF":fxp<+/-,17,17>)
      }
    }
    n229 = Greater?(x=w64, y=39) -> (0:w62:bool)
    n230 = Greater?(x=w64, y=38) -> (0:w72:bool)
    n231 = Select(t=1, s=w72, f=0) -> (s? t:f=w70:i32)
    n232 = Select(t=1, s=w62, f=0) -> (s? t:f=w67:i32)
  }
  n233 = while {
    tunnel: w1 -> [w856]
    i -> [w855]
    stop <- "stop 2" stop-if-true
    # "2."
    n234 = xnode "FPGA I/O Method Node"("error in"=w856, "Timeout"=41000000) -> ("error out"=w861:errorcluster, "Timed Out"=w858:bool)  [unwired: 1 in, 1 out]
    "Timed Out" <- w858
    n235 = case shown="False" w858 {
      tunnel: w861 -> [w876 w877]
      tunnel: [w865 w877] -> w860
      frame False {
        # "3."
        n236 = xnode "FPGA I/O Property Node"("error in"=w876) -> ("error out"=w865:errorcluster, "PPS Timestamp (TAI)"=→"PPS Timestamp (TAI)":u64, "UTC Offset"=→"UTC Offset":i8, "UTC Offset Valid"=→"UTC Offset Valid":bool, "GPS Status"=→"GPS Status":T1, "Antenna Status"=→"Antenna Status":T2, "Leap Second Direction"=→"Leap Second Direction":enum8{"Add", "Delete"}, "Leap Second Pending"=→"Leap Second Pending":bool, "Leap Second Occurred"=→"Leap Second Occurred":bool, "Satellites Available"=→"Satellites Available":u8, "Self-Survey Complete"=→"Self-Survey Complete":bool, "Latitude (°)"=→"Latitude (°)":T3, "Longitude (°)"=→"Longitude (°)":T4, "Altitude (m)"=→"Altitude (m)":T5)  [unwired: 1 in, 1 out]
      }
      frame True {
      }
    }
    "FPGA Error Out" <- w860
    "Iterations" <- w855
  }
  n237 = while {
    stop <- FALSE stop-if-true
    # "2. Update the FPGA Timekeeper time indicator."
    n238 = call "Get Time.vi"() -> ("time (ns)"=→"FPGA Timekeeper time (ns) 2":u64)
  }
